vi "Format Header.vi"(5 "Name":string[](array[string]), 7 "Value":string[](array[string]), 11 "XML in":refnum<class "XML.lvclass">) -> (3 "XML out":refnum<class "XML.lvclass">, 4 "Header":string)   [LabVIEW 2020, in "XML.lvlib" / "XML.lvclass"]
uses:
  <vilib>/gpm_packages/@cs/persistence/source/XML/XML.lvclass
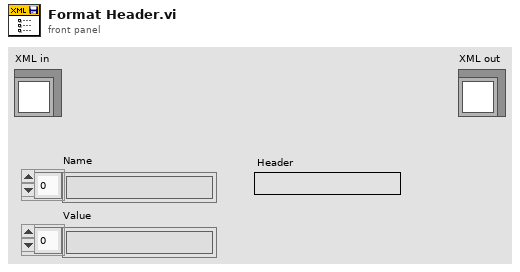
[diagram p1: front panel]
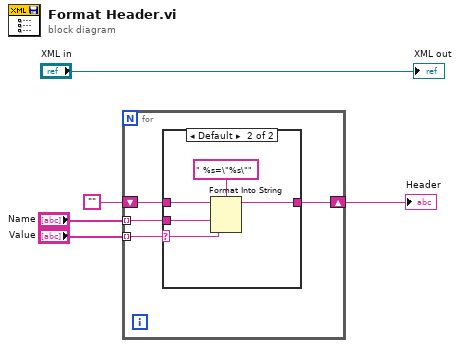
[diagram p0: block diagram]
diagram:
  n1 = for {
    tunnel: "Name" -> [w9] mode=indexing
    tunnel: "Value" -> [w8] mode=indexing
    shift-right: [w6] -> w1
    shift-left: "" -> [w7]
    n2 = case shown="Default" w8 {
      selector: w8 -> [_ w13]
      tunnel: w9 -> [_ w14]
      tunnel: w7 -> [w10 w12]
      tunnel: [w10 w11] -> w6
      frame "" {
      }
      frame Default {
        n3 = Format Into String(format string=" %s=\"%s\"", initial string=w12, w14, w13) -> (resulting string=w11:string)  [unwired: 1 in, 1 out]
      }
    }
  }
  "Header" <- w1
  "XML out" <- "XML in"
